vi "Configure OSC Limit Short query.vi"(8 "error in (no error)":errorcluster, 10 "Step":T1=1 min=1 max=99 step=1, 11 "VISA resource name":refnum<visa-resource-name>) -> (0 "error out":errorcluster, 2 "Limit short":string, 3 "VISA resource name out":refnum<visa-resource-name>)   [LabVIEW 2025, in "Chroma 19052.lvlib"]
uses:
  <instrlib>/Chroma 19052/Public/Utility/Type Def/steps--numeric.ctl
  <instrlib>/Chroma 19052/Chroma 19052.lvlib
panel:
  # "OSC Limit Short query"
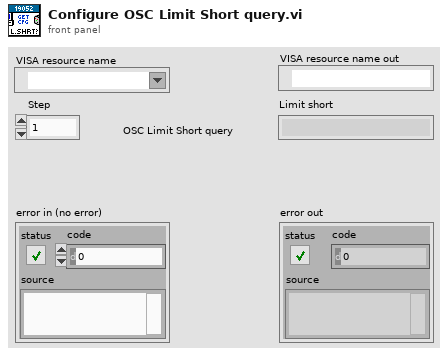
[diagram p1: front panel]
types:
  T1 = typedef "Chroma 19052.lvlib/steps--numeric.ctl" = u8
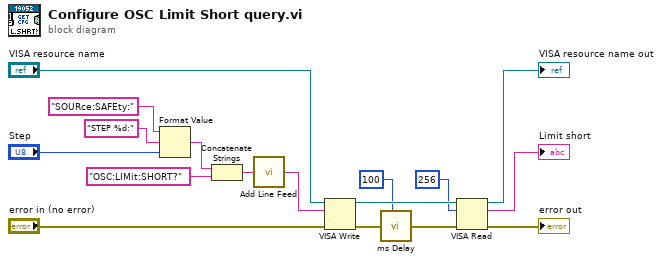
[diagram p0: block diagram]
diagram:
  n1 = Format Value(string ("")="SOURce:SAFEty:", format string="STEP %d:", value (0)="Step") -> (output string=w1:string)
  n2 = Concatenate Strings(w1, "OSC:LIMit:SHORT?" ("format string")) -> (w11:string)
  n3 = call <instrlib>:"Add Line Feed.vi"("Command string"=w11) -> ("Concatenated string"=w9:string)  [unwired: 4 in]
  n4 = VISA Write(VISA resource name="VISA resource name", write buffer=w9, error in (no error)="error in (no error)") -> (VISA resource name out=w17:refnum<visa-resource-name>, error out=w6:errorcluster)  [unwired: 1 out]
  n5 = call <instrlib>:"ms Delay.vi"("miliseconds to wait"=u32 100 ("Time Delay ms"), "error in (no error)"=w6) -> ("error out"=w5:errorcluster)  [unwired: 6 in, 1 out]
  n6 = VISA Read(VISA resource name=w17, byte count=u32 256, error in (no error)=w5) -> (VISA resource name out=→"VISA resource name out":refnum<visa-resource-name>, read buffer=→"Limit short":string, error out=→"error out":errorcluster)  [unwired: 1 out]
